vi "FalseColor.vi"(0 "Black zero":bool, 1 "Palette Number (gray)":T2(ring)=enum."Temperature", 5 "Image":T1, 7 "Image Dst":T1, 9 "Operator":T3(ring)=enum."Clear  if > or =", 11 "error in (no error)":errorcluster) -> (6 "Image Dst Out":T1, 10 "error out":errorcluster)   [LabVIEW 2014]
uses:
  <vilib>/vision/Image Controls.llb/IMAQ Image.ctl
  <vilib>/vision/NI_Vision_Development_Module.lvlib
panel:
  out "Color Palette":cluster{"Red":u8, "Green":u8, "Blue":u8}[](array[cluster])
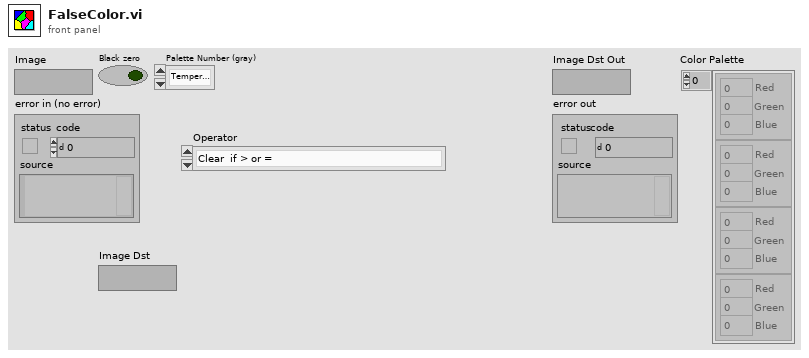
[diagram p1: front panel]
types:
  T1 = typedef "IMAQ Image.ctl" = refnum<image>
  T2 = enum32{"Gray", "Binary", "Gradient", "Rainbow", "Temperature"}
  T3 = enum32{"Average", "Min", "Max", "Clear  if < ", "Clear  if < or =", "Clear  if =", "Clear  if > or =", "Clear  if >"}
  T4 = typedef "Image Type" = u32
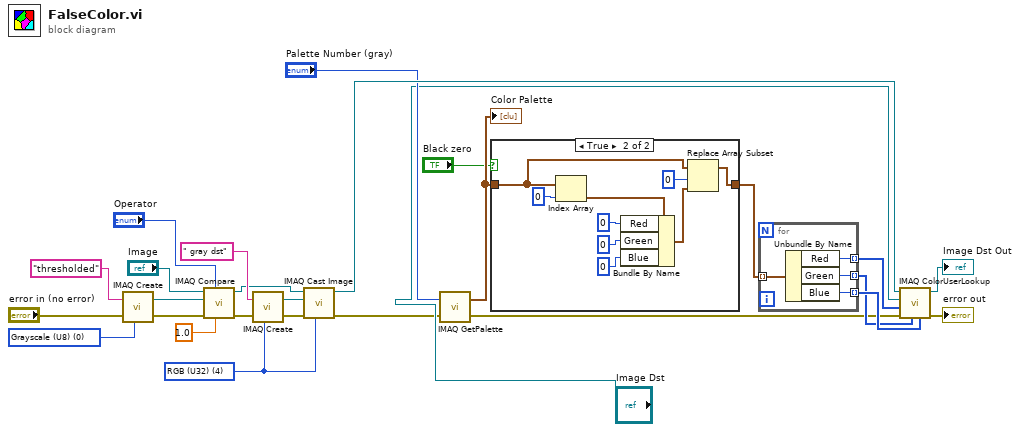
[diagram p0: block diagram]
diagram:
  w5 = T4 0 items=["Grayscale (U8)", "Grayscale (I16)", "Grayscale (SGL)", "Complex (CSG)", "RGB (U32)", "HSL (U32)", "RGB (U64)", "Grayscale (U16)"] ("Image Type")
  w17 = T4 4 items=["Grayscale (U8)", "Grayscale (I16)", "Grayscale (SGL)", "Complex (CSG)", "RGB (U32)", "HSL (U32)", "RGB (U64)", "Grayscale (U16)"] ("Image Type")
  n1 = call "IMAQ Create"("Image Name"="thresholded", "Image Type"=w5, "error in (no error)"="error in (no error)") -> ("New Image"=w20:T1, "error out"=w14:errorcluster)  [unwired: 2 in]
  n2 = call "IMAQ Compare"("Constant"=1.0 ("x"), "Operator"="Operator", "error in (no error)"=w14, "Image Dst"=w20, "Image Src A"="Image") -> ("error out"=w13:errorcluster, "Image Dst Out"=w19:T1)  [unwired: 5 in]
  n3 = call "IMAQ Create"("Image Name"=" gray dst", "Image Type"=w17, "error in (no error)"=w13) -> ("New Image"=w23:T1, "error out"=w12:errorcluster)  [unwired: 1 in, 1 out]
  n4 = call "IMAQ Cast Image"("Image Type"=w17, "error in (no error)"=w12, "Image Dst"=w23, "Image Src"=w19) -> ("error out"=w1:errorcluster, "Image Dst Out"=w22:T1)  [unwired: 6 in]
  n5 = call "IMAQ GetPalette"("Palette Number (gray)"="Palette Number (gray)", "error in (no error)"=w1) -> ("Color Palette"=w8:cluster{"Red":u8, "Green":u8, "Blue":u8}[], "error out"=w11:errorcluster)  [unwired: 3 in]
  "Color Palette" <- w8
  n6 = case shown="True" "Black zero" {
    tunnel: w8 -> [w28 w36]
    tunnel: [w28 w29] -> w6
    frame False {
    }
    frame True {
      n7 = Index Array(array=w36, index=0) -> (element=w34:cluster{"Red":u8, "Green":u8, "Blue":u8})
      n8 = Bundle By Name(cluster=w34, "Red"=u8 0, "Green"=u8 0, "Blue"=u8 0) -> (w30:cluster{"Red":u8, "Green":u8, "Blue":u8})
      n9 = Replace Array Subset(array=w36, new element=w30, index=0) -> (w29:cluster{"Red":u8, "Green":u8, "Blue":u8}[])
    }
  }
  n10 = for {
    tunnel: w6 -> [w41] mode=indexing
    tunnel: [w40] -> w25 mode=indexing
    tunnel: [w39] -> w26 mode=indexing
    tunnel: [w38] -> w27 mode=indexing
    n11 = Unbundle By Name(w41) -> ("Red"=w40:u8, "Green"=w39:u8, "Blue"=w38:u8)
  }
  n12 = call "IMAQ ColorUserLookup"("Blue or Luma or Val or Inten Lookup Table"=w27, "Green or Sat Lookup Table"=w26, "error in (no error)"=w11, "Red or Hue Lookup Table"=w25, "Image Dst"="Image Dst", "Image Src"=w22) -> ("error out"=→"error out":errorcluster, "Image Dst Out"=→"Image Dst Out":T1)  [unwired: 4 in]
